vi "RGBA to 3D Array.vi"(0 "24-bit pixmap":u32[][](array[numeric]), 1 "Keep Alpha":bool) -> (2 "RGB Array":u8[][][](array[numeric]))   [LabVIEW 2020, in "LV Tiff.lvlib"]
uses:
  LV Tiff.lvlib
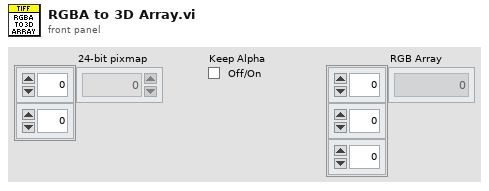
[diagram p1: front panel]
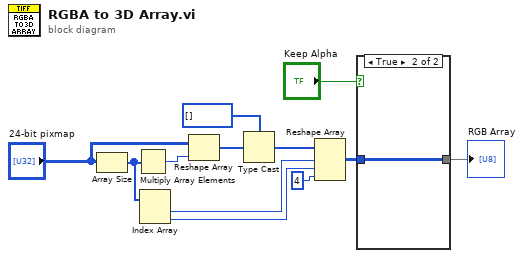
[diagram p0: block diagram]
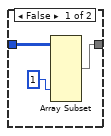
[diagram p2: hidden frame]
diagram:
  n1 = Array Size(array="24-bit pixmap") -> (size(s)=w6:i32[])
  n2 = Multiply Array Elements(1:w6) -> (0:w2:i32)
  n3 = Index Array(array=w6) -> (element #1=w9:i32, element #2=w10:i32)  [unwired: 2 in]
  n4 = Reshape Array("24-bit pixmap", w2) -> (w3:u32[])
  n5 = Type Cast(type=u8[] [], x=w3) -> (*(type *) &x=w5:u8[])
  n6 = Reshape Array(w5, w9, w10, 4 ("dimension size")) -> (w7:u8[][][])
  n7 = case shown="True" "Keep Alpha" {
    tunnel: [w15 w16] -> w12
    tunnel: w7 -> [w13 w16]
    frame False {
      n8 = Array Subset(array=w13, index (dim 2)=1 ("index")) -> (w15:u8[][][])  [unwired: 5 in]
    }
    frame True {
    }
  }
  "RGB Array" <- w12
